vi "Main.vi"() -> ()   [LabVIEW 2019]
uses:
  States.ctl
  Operations.ctl
  <vilib>/ErrorRing/Error Ring.xnode
panel:
  in  "Buttons":T1
  out "Display":string
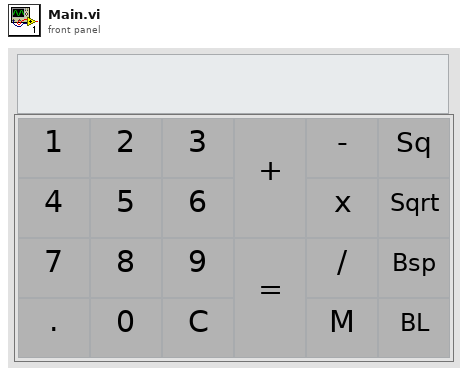
[diagram p1: front panel]
types:
  T1 = cluster{"1":bool, "2":bool, "3":bool, "4":bool, "5":bool, "6":bool, "7":bool, "8":bool, "9":bool, "0":bool, "Clear":bool, "Dot":bool, "Add":bool, "Equal":bool, "Sub":bool, "Mult":bool, "Div":bool, "Memory":bool, "Square":bool, "Sqrt":bool, "BackSpace":bool, "BackLight":bool}
  T2 = typedef "States.ctl" = enum16{"Idle", "DataIntialize", "UIInitialize", "UIUpdate", "Operation", "NextNumber", "Exit"}
  T3 = typedef "Operations.ctl" = enum16{"Add", "NoOp", "Sub", "Mult", "Div", "Sqrt", "Square", "Dot", "Clear", "BackSpace", "Memory"}
  T4 = cluster{"TimeOut":i32, "Number":string, "NexNumber":string[], "Ops":T3, "Result":string}
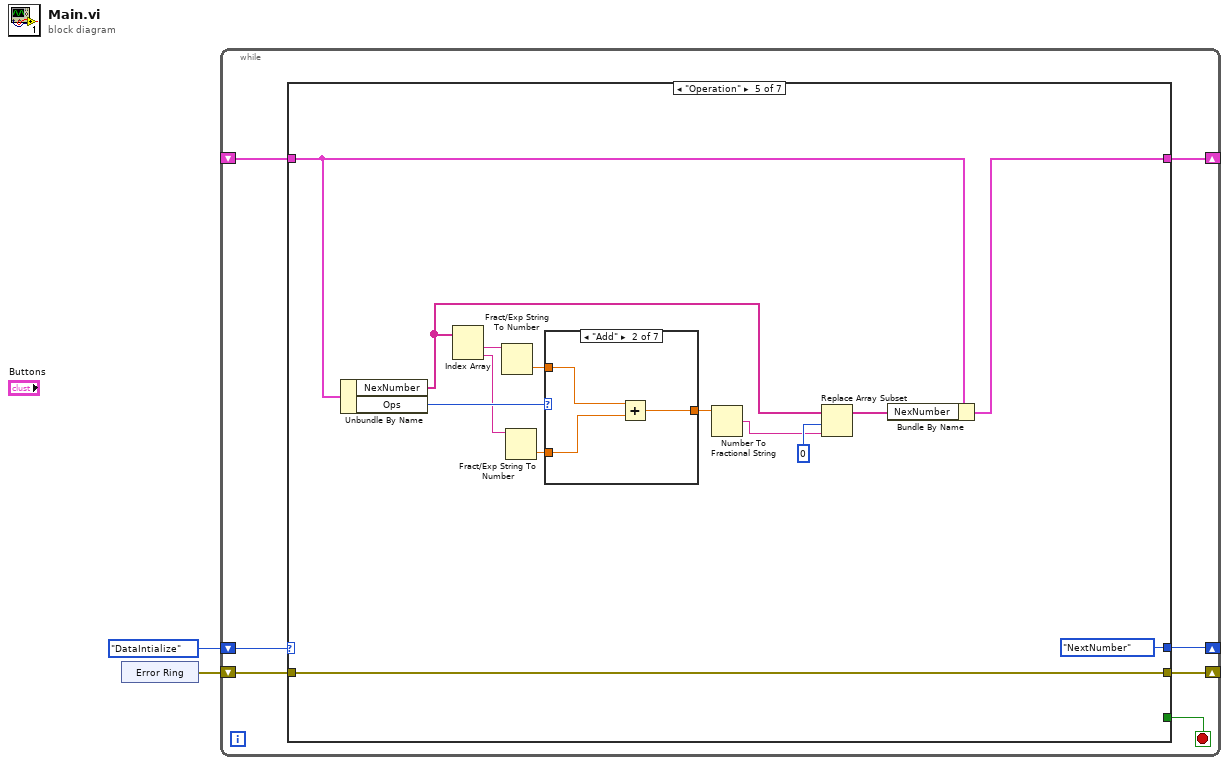
[diagram p0: block diagram]
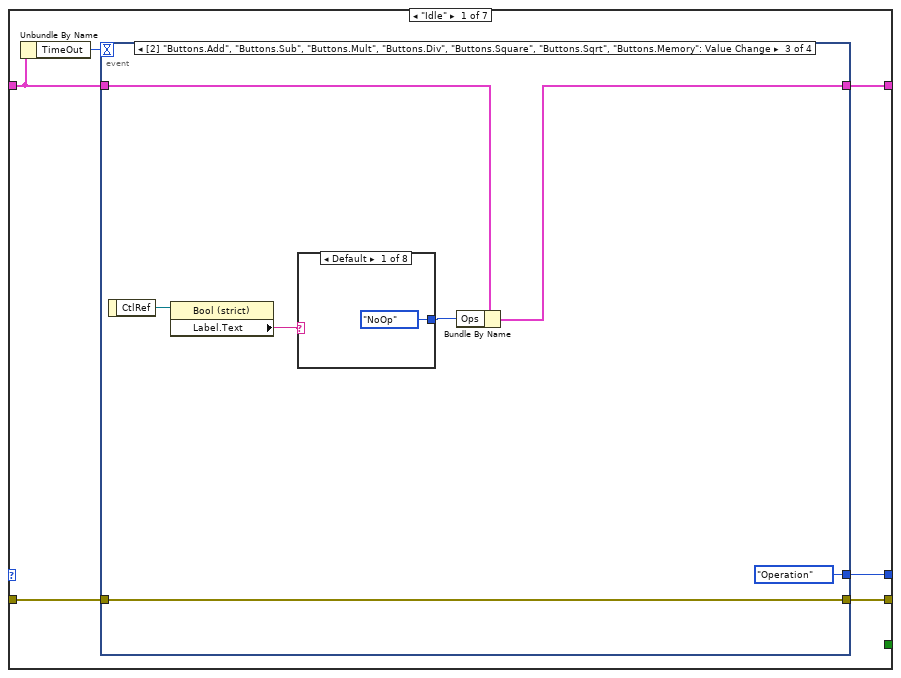
[diagram p2: hidden frame]
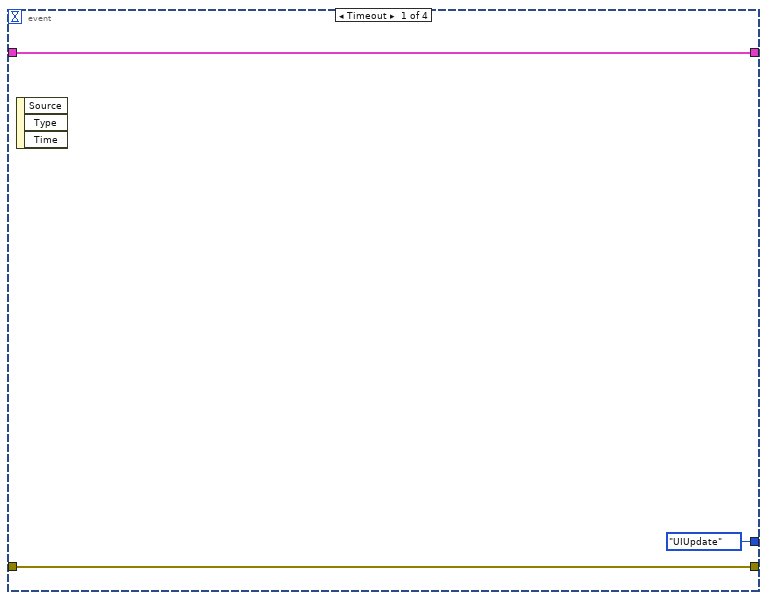
[diagram p3: hidden frame]
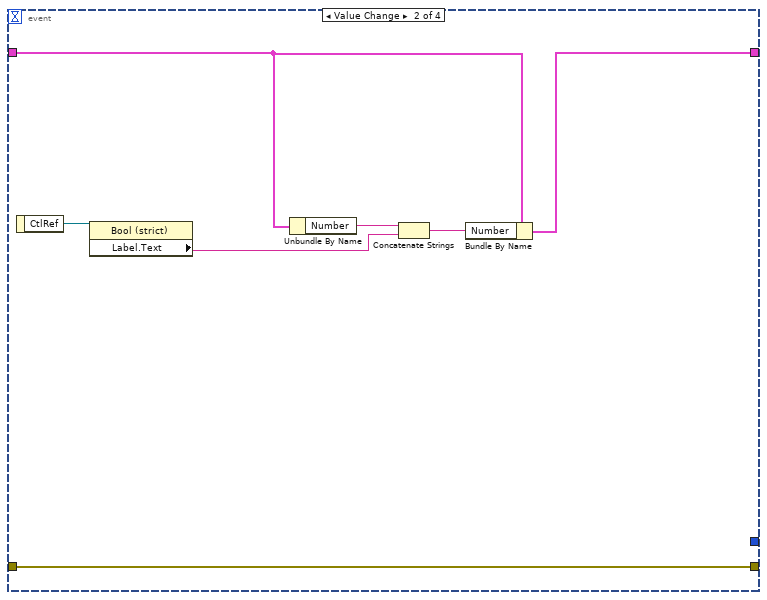
[diagram p4: hidden frame]
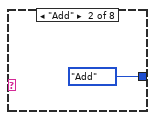
[diagram p5: hidden frame]
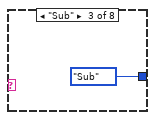
[diagram p6: hidden frame]
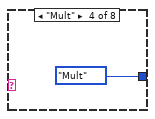
[diagram p7: hidden frame]
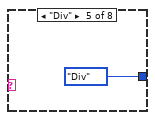
[diagram p8: hidden frame]
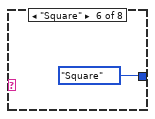
[diagram p9: hidden frame]
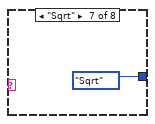
[diagram p10: hidden frame]
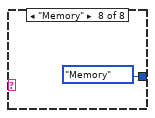
[diagram p11: hidden frame]
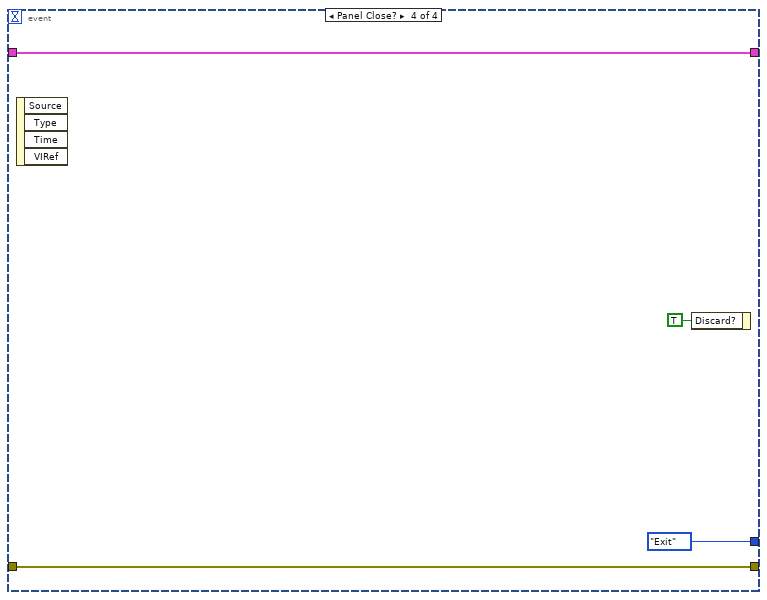
[diagram p12: hidden frame]
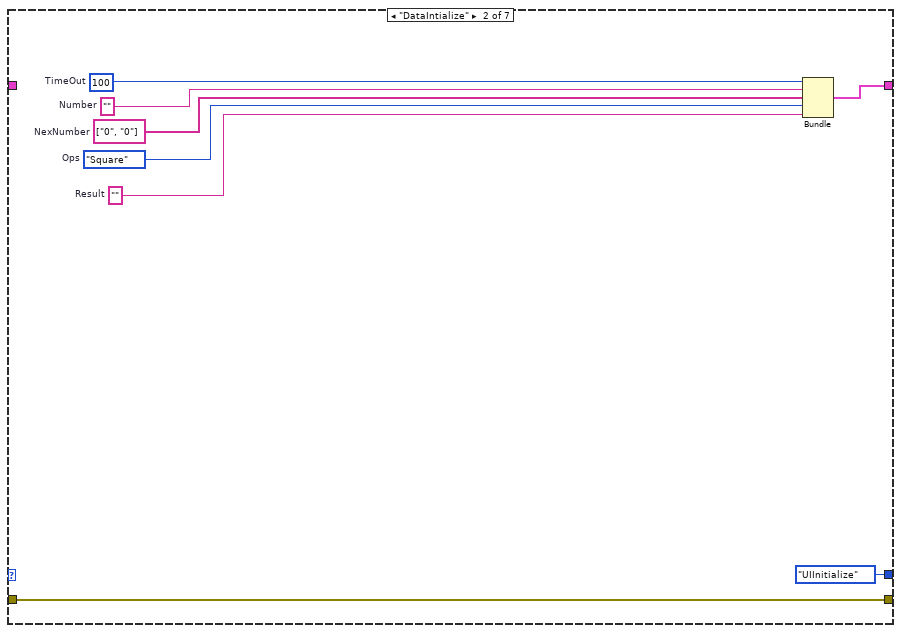
[diagram p13: hidden frame]
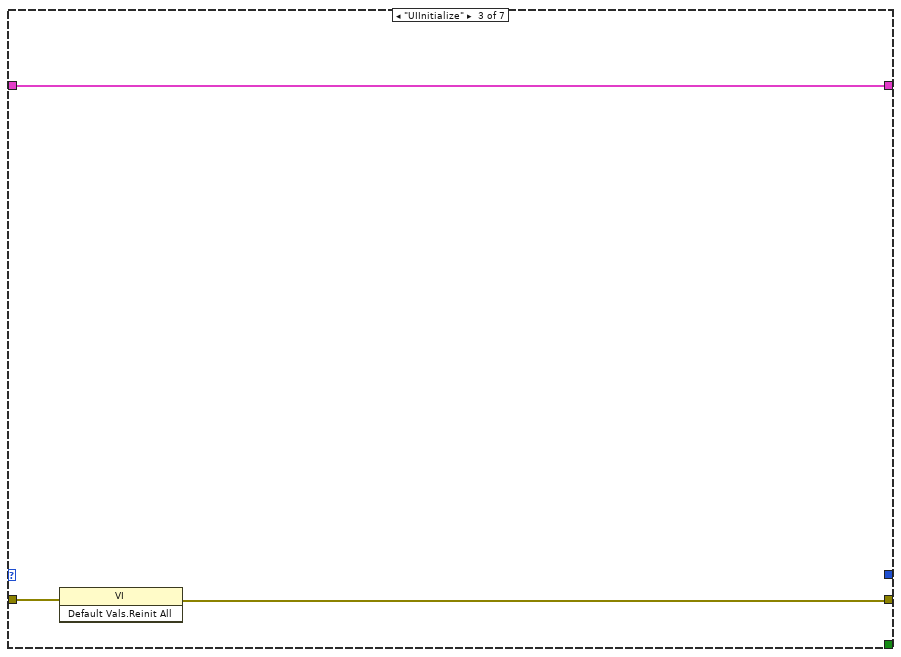
[diagram p14: hidden frame]
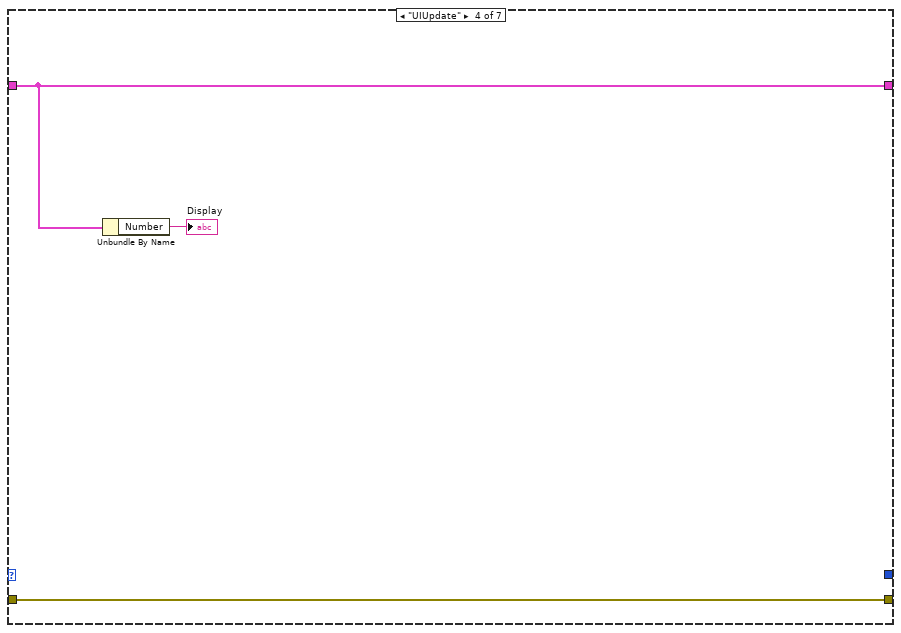
[diagram p15: hidden frame]
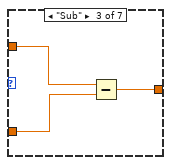
[diagram p17: hidden frame]
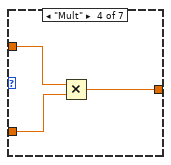
[diagram p18: hidden frame]
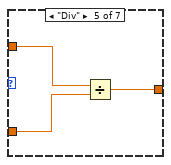
[diagram p19: hidden frame]
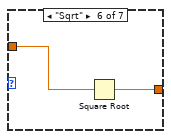
[diagram p20: hidden frame]
diagram:
  n1 = xnode "Error Ring"() -> ("error out"=w1:errorcluster)
  n2 = while {
    shift-right: [w3] -> _
    shift-left: States."DataIntialize" ("States") -> [w9]
    shift-right: [w7] -> _
    shift-left: w1 -> [w8]
    shift-right: [w6] -> _
    shift-left: _ -> [w5]
    stop <- w4 stop-if-true
    n3 = case shown="\"Operation\"" w9 {
      tunnel: w8 -> [w15 w52 w54 w58 w72 w97 w100]
      tunnel: [w14 w52 w53 w58 w72 w97 w100] -> w7
      tunnel: [w13 w51 w55 w57 w65 w96 w99] -> w6
      tunnel: w5 -> [w11 _ w55 w57 w64 w95 w99]
      tunnel: [_ _ _ _ _ _ TRUE] -> w4
      tunnel: [w12 States."UIInitialize" ("States") _ _ States."NextNumber" ("States") _ _] -> w3
      frame "Idle" {
        n4 = Unbundle By Name(w11) -> ("TimeOut"=w10:i32)
        n5 = event shown="[2] \"Buttons.Add\", \"Buttons.Sub\", \"Buttons.Mult\", \"Buttons.Div\", \"Buttons.Square\", \"Buttons.Sqrt\", \"Buttons.Memory\": Value Change" {
          selector: _ -> [_ _ _ _]
          dyn-events: _ -> [_ _ _ _]
          timeout: w10 -> [_ _ _ _]
          tunnel: w15 -> [w18 w25 w32 w44]
          tunnel: [w18 w25 w32 w44] -> w14
          tunnel: w11 -> [w17 w22 w27 w43]
          tunnel: [w17 w23 w28 w43] -> w13
          tunnel: [States."UIUpdate" ("States") _ States."Operation" ("States") States."Exit" ("States")] -> w12
          event Timeout {
            n6 = event-data() -> ()  [unwired: 1 in, 3 out]
          }
          event "Buttons.1", "Buttons.2", "Buttons.3", "Buttons.4", "Buttons.5", "Buttons.6", "Buttons.7", "Buttons.8", "Buttons.9", "Buttons.0": Value Change {
            n7 = event-data() -> ("CtlRef"=w24:refnum<vi>)  [unwired: 1 in]
            n8 = property class="Bool (strict)"(reference=w24) -> ("Label.Text"=w20:string)  [unwired: 1 in, 2 out]
            n9 = Unbundle By Name(w22) -> ("Number"=w21:string)
            n10 = Concatenate Strings(w21, w20) -> (w19:string)
            n11 = Bundle By Name(cluster=w22, "Number"=w19) -> (w23:T4)
          }
          event "Buttons.Add", "Buttons.Sub", "Buttons.Mult", "Buttons.Div", "Buttons.Square", "Buttons.Sqrt", "Buttons.Memory": Value Change {
            n12 = event-data() -> ("CtlRef"=w31:refnum<vi>)  [unwired: 1 in]
            n13 = property class="Bool (strict)"(reference=w31) -> ("Label.Text"=w30:string)  [unwired: 1 in, 2 out]
            n14 = case shown="Default" w30 {
              tunnel: [Operations."NoOp" ("Ops") Operations."Add" ("Ops") Operations."Sub" ("Ops") Operations."Mult" ("Ops") Operations."Div" ("Ops") Operations."Square" ("Ops") Operations."Sqrt" ("Ops") Operations."Memory" ("Ops")] -> w29
              frame Default {
              }
              frame "Add" {
              }
              frame "Sub" {
              }
              frame "Mult" {
              }
              frame "Div" {
              }
              frame "Square" {
              }
              frame "Sqrt" {
              }
              frame "Memory" {
              }
            }
            n15 = Bundle By Name(cluster=w27, "Ops"=w29) -> (w28:T4)
          }
          event Panel Close? {
            n16 = event-data() -> ()  [unwired: 1 in, 4 out]
            n17 = event-data("Discard?"=TRUE) -> ()  [unwired: 1 in, 1 out]
          }
        }
      }
      frame "DataIntialize" {
        w45 = ""  # Result
        w47 = Operations."Square"  # Ops
        w48 = string[] ["0", "0"]  # NexNumber
        w49 = ""  # Number
        w50 = 100  # TimeOut
        n18 = Bundle("TimeOut"=w50, "Number"=w49, "NexNumber"=w48, "Ops"=w47, "Result"=w45) -> (w51:T4)  [unwired: 1 in]
      }
      frame "UIInitialize" {
        n19 = invoke class="VI" method="Default Vals.Reinit All"(error in=w54) -> (error out=w53:errorcluster)  [unwired: 2 in, 2 out]
      }
      frame "UIUpdate" {
        n20 = Unbundle By Name(w57) -> ("Number"=→"Display":string)
      }
      frame "Operation" {
        n21 = Unbundle By Name(w64) -> ("NexNumber"=w62:string[], "Ops"=w71:T3)
        n22 = Index Array(array=w62) -> (element #1=w70:string, element #2=w69:string)  [unwired: 2 in]
        n23 = Fract/Exp String To Number(string=w70) -> (number=w68:dbl)  [unwired: 3 in, 1 out]
        n24 = Fract/Exp String To Number(string=w69) -> (number=w67:dbl)  [unwired: 3 in, 1 out]
        n25 = case shown="\"Add\"" w71 {
          tunnel: w68 -> [_ w75 w78 w81 w84 w86 w88]
          tunnel: w67 -> [_ w74 w77 w80 w83 _ _]
          tunnel: [_ w73 w76 w79 w82 w85 w87] -> w66
          frame "NoOp", Default {
          }
          frame "Add" {
            n26 = Add(x=w75, y=w74) -> (x+y=w73:dbl)
          }
          frame "Sub" {
            n27 = Subtract(x=w78, y=w77) -> (x-y=w76:dbl)
          }
          frame "Mult" {
            n28 = Multiply(x=w81, y=w80) -> (x*y=w79:dbl)
          }
          frame "Div" {
            n29 = Divide(x=w84, y=w83) -> (x/y=w82:dbl)
          }
          frame "Sqrt" {
            n30 = Square Root(x=w86) -> (sqrt(x)=w85:dbl)
          }
          frame "Square" {
            n31 = Square(x=w88) -> (x^2=w87:dbl)
          }
        }
        n32 = Number To Fractional String(number=w66) -> (F-format string=w60:string)  [unwired: 3 in]
        n33 = Replace Array Subset(array=w62, new element=w60, index=0) -> (w59:string[])
        n34 = Bundle By Name(cluster=w64, "NexNumber"=w59) -> (w65:T4)
      }
      frame "NextNumber" {
        n35 = Unbundle By Name(w95) -> ("NexNumber"=w94:string[], "Number"=w89:string, "Result"=w91:string)
        n36 = Replace Array Subset(array=w94, new element #1=w89, index #1=0 ("index"), new element #2=w91, index #2=1 ("index")) -> (w90:string[])
        n37 = Bundle By Name(cluster=w95, "NexNumber"=w90, "Number"=w89) -> (w96:T4)
      }
      frame "Exit" {
      }
    }
  }
